vi "Do.vi"(8 "error in (no error)":errorcluster, 10 "Actor in":refnum<class "Actor.lvclass">, 11 "Send Run Measurement Message":refnum<class "Send Run Measurement Message.lvclass">) -> (0 "error out":errorcluster, 2 "Actor out":refnum<class "Actor.lvclass">)   [LabVIEW 2017, in "Measurement UI.lvlib" / "Send Run Measurement Message.lvclass"]
uses:
  Send Run Measurement Message.lvclass
  <vilib>/ActorFramework/Actor/Actor.lvclass
  Measurement UI.lvclass
  C:/Program Files (x86)/National Instruments/LabVIEW 2017/vi.lib/ActorFramework/Actor/Actor.lvclass
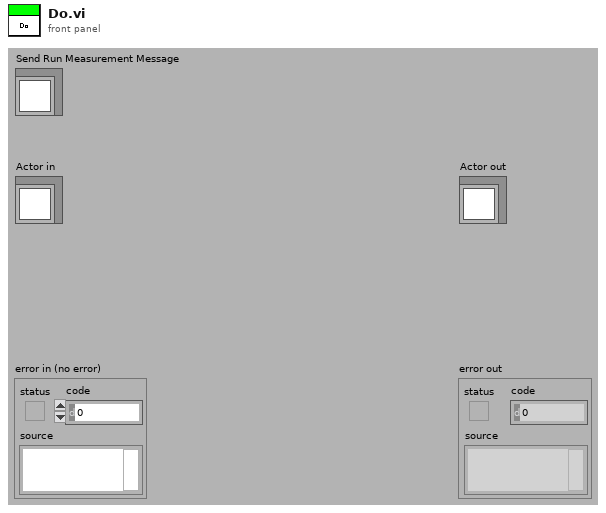
[diagram p1: front panel]
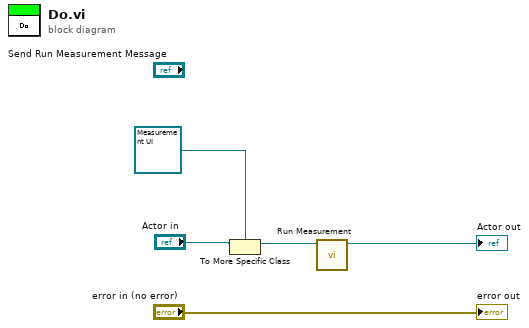
[diagram p0: block diagram]
diagram:
  n1 = To More Specific Class(target class=refnum<class "Measurement UI.lvclass"> refnum ("UI.lvclass"), reference="Actor in") -> (specific class reference=w2:refnum<class "Measurement UI.lvclass">)  [unwired: 1 in, 1 out]
  n2 = call-dynamic "Run Measurement.vi"("Operator UI in"=w2) -> ("Operator UI out"=→"Actor out":refnum<class "Measurement UI.lvclass">)  [unwired: 9 in, 1 out]
  "error out" <- "error in (no error)"
